vi "Write configuration.vi"(8 "error in":errorcluster, 10 "configuration":refnum<class "NISE_CEF_serializable configuration.lvclass">, 11 "fixed channel editor in":refnum<class "fixed channel editor.lvclass">) -> (0 "error out":errorcluster, 3 "fixed channel editor out":refnum<class "fixed channel editor.lvclass">)   [LabVIEW 2013, in "fixed channel editor.lvclass"]
uses:
  fixed channel editor.lvclass
  module/configuration/fixed channel configuration.lvclass
  <vilib>/NI/Configuration Framework/serializable configuration/NISE_CEF_serializable configuration.lvclass
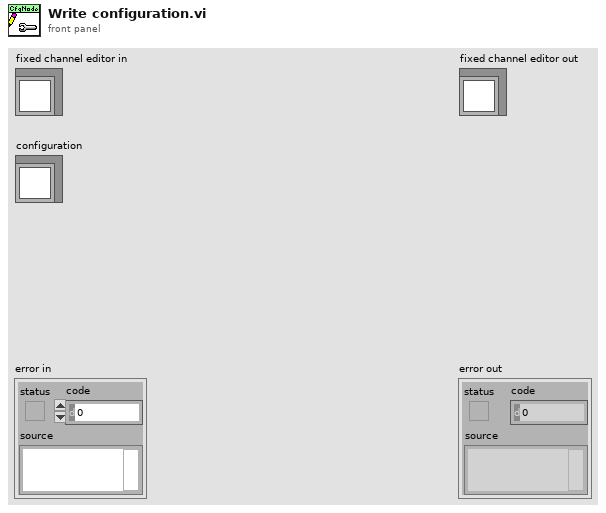
[diagram p1: front panel]
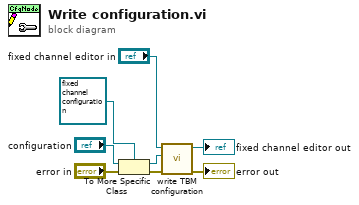
[diagram p0: block diagram]
diagram:
  n1 = To More Specific Class(target class=refnum<class "fixed channel configuration.lvclass"> refnum ("fixed channel configuration"), reference="configuration", error in="error in") -> (specific class reference=w1:refnum<class "fixed channel configuration.lvclass">, error out=w4:errorcluster)
  n2 = call-dynamic "write TBM configuration.vi"("error in"=w4, "configuration"=w1, "fixed module parent implementation editor node in"="fixed channel editor in") -> ("error out"=→"error out":errorcluster, "fixed module parent implementation editor node out"=→"fixed channel editor out":refnum<class "fixed channel editor.lvclass">)  [unwired: 7 in]
